vi "Main Tclk.vi"() -> ()   [LabVIEW 2018] (continued)
          tunnel: w2699 -> [w3069 _]
          frame False {
            n3729 = case shown="\"SEM Low Mag Scan\"" w3069 {
              tunnel: w3070 -> [w3073 w3074]
              tunnel: w3071 -> [w3072 w3075]
              frame Default {
                "Detector B" <- w3073
                "Detector A" <- w3072
              }
              frame "SEM Low Mag Scan" {
                "Detector A Low Mag" <- w3075
                "Det A LM" <- w3075
                "Detector B Low Mag" <- w3074
                "Det B LM" <- w3074
              }
            }
          }
          frame True {
            n3730 = shared-variable "My Computer\\Zeiss Library.lvlib\\DetA-scaling"() -> (→"DetA e- Scaling":sgl)  [unwired: 1 in, 1 out]
            n3731 = shared-variable "My Computer\\Zeiss Library.lvlib\\DetB-Scaling"() -> (→"DetB e- Scaling":sgl)  [unwired: 1 in, 1 out]
          }
        }
        n3732 = case shown="False" w2775 {
          tunnel: w2774 -> [w3056 _]
          frame False {
            n3733 = Build Array("Pre image", "Post image") -> (w3058:bool[])
            n3734 = Boolean Array To Number(Boolean array=w3058) -> (number=w3057:u32)
            n3735 = case shown="0, Default" w3057 {
              tunnel: w3056 -> [w3061 w3062 w3063]
              frame 0, Default {
                "FIB Image" <- w3061
              }
              frame 1 {
                "Pre Image" <- w3062
              }
              frame 2 {
                "Post Image" <- w3063
              }
            }
          }
          frame True {
          }
        }
        n3736 = In Range and Coerce(upper limit=w2637, x=w2638, lower limit=sgl 0.0) -> (coerced(x)=w2635:sgl)  [unwired: 1 out]
        n3737 = shared-variable ".\\Zeiss Library.lvlib\\Det"(w2802) -> ()  [unwired: 1 in, 1 out]
        n3738 = Add(x=w2814, y=w2813) -> (x+y=w2812:u16)
        n3739 = Bundle By Name(cluster=w2636, "Focus index stop limit"=w2635) -> (w2634:T36)
        n3740 = Equal To 0?(x=w2812) -> (x = 0?=w2810:bool)
        n3741 = Divide(x=w2715, y=w2711) -> (x/y=w2714:sgl)
        n3742 = Increment(x=w2827) -> (x+1=w2823:sgl)
        n3743 = Divide(x=w2712, y=w2711) -> (x/y=w2713:sgl)
        n3744 = To Double Precision Float(number=w2826) -> (double precision float=w2825:dbl)
        n3745 = Reciprocal(x=w2825) -> (1/x=w2824:dbl)
        n3746 = Multiply(x=w2714, y=w2823) -> (x*y=w2821:sgl)
        n3747 = Multiply(x=w2714, y=w2713) -> (x*y=w2822:sgl)
        n3748 = And(x=w2811, y=w2810) -> (x .and. y?=w2809:bool)
        n3749 = local read "Load recipe"() -> (w2632:bool)
        n3750 = Divide(x=w2822, y=w2623) -> (x/y=w2626:sgl)
        n3751 = Compound Arithmetic op=MULTIPLY(w2629, w2824, w2821, w2713) -> (w2829:dbl)
        "SEM scan time" <- w2829
        n3752 = local read "Detector number"() -> (w2643:i16)
        n3753 = property on="Total pixels recorded" class="Slide (strict)"("Scale.Maximum"=w2626) -> ()  [unwired: 2 in, 2 out]
        n3754 = Quotient & Remainder(x=w2829, y=60.0) -> (x-y*floor(x/y)=w2831:dbl, floor(x/y)=w2832:dbl)
        n3755 = To Variant(anything="FIB Scan Parameters") -> (Variant=w2803:variant)
        n3756 = local read "SEM Status"() -> (w2830:T12)
        n3757 = case shown="Default" w2699 {
          frame "SEM Low Mag Scan" {
          }
          frame Default {
            n3758 = shared-variable ".\\Zeiss Library.lvlib\\Det A Img Tiled"() -> (→"Det A":i16[][])  [unwired: 1 in, 1 out]
            n3759 = shared-variable ".\\Zeiss Library.lvlib\\Det B Img Tiled"() -> (→"Det B":i16[][])  [unwired: 1 in, 1 out]
          }
        }
        n3760 = Bundle By Name(cluster=w2830, "Scan time (s)"=w2831, "Scan time (m)"=w2832, "Detector #"=w2643) -> (w2818:T12)
        n3761 = case shown="False" w2632 {
          tunnel: w2634 -> [_ w2845]
          frame False {
          }
          frame True {
            n3762 = local write "Alert Settings"(w2845) -> ()
          }
        }
        n3763 = shared-variable ".\\Zeiss Library.lvlib\\Realtime Imaging Scan Para"(w2803) -> ()  [unwired: 1 in, 1 out]
        n3764 = To Variant(anything=w2818) -> (Variant=w2817:variant)
        n3765 = case shown="False" w2809 {
          tunnel: w2818 -> [_ w3120]
          tunnel: w2817 -> [_ w3119]
          tunnel: w2807 -> [w3118 _]
          frame False {
            "SEM Status" <- w3118
          }
          frame True {
            n3766 = shared-variable ".\\Zeiss Library.lvlib\\SEMInfo"(w3119) -> ()  [unwired: 2 out]
            n3767 = local write "SEM Status"(w3120) -> ()
          }
        }
        n3768 = local read "Low Mag SEM"() -> (w2670:T30)
        n3769 = local read "SEM Low Mag Scan Parameters"() -> (w2669:T5)
        n3770 = local read "SEM Mid Mag Scan Parameters"() -> (w2668:T5)
        n3771 = Unbundle By Name(w2670) -> ("Low mag scan"=w2753:bool, "Show HM box"=w2773:bool)
        n3772 = property on="Sweep direction" class="Bool (strict)"("Visible"="Sweep enabled") -> ()  [unwired: 2 in, 2 out]
        n3773 = property on="Sweep rate (Hz)" class="DigNum (strict)"("Visible"="Sweep enabled") -> ()  [unwired: 2 in, 2 out]
        n3774 = property on="Level #" class="DigNum (strict)"("Visible"="Sweep enabled") -> ()  [unwired: 2 in, 2 out]
        n3775 = property on="Sweep #" class="DigNum (strict)"("Visible"="Sweep enabled") -> ()  [unwired: 2 in, 2 out]
        n3776 = local read "Milling para"() -> (w2641:T35)
        n3777 = shared-variable ".\\Zeiss Library.lvlib\\FIB PID reset"() -> (w2640:bool)  [unwired: 1 in, 1 out]
        n3778 = local read "Milling para"() -> (w2738:T35)
        n3779 = Unbundle By Name(w2669) -> ("Scan rate (Hz)"=w2671:u32, "X size (um)"=w2675:sgl, "Y size (um)"=w2679:sgl, "Pixel size (nm)"=w2674:sgl)
        n3780 = Unbundle By Name(w2668) -> ("Scan rate (Hz)"=w2741:u32, "X size (um)"=w2709:sgl, "Y size (um)"=w2705:sgl, "Pixel size (nm)"=w2710:sgl)
        n3781 = case shown="False" w2753 {
          tunnel: [T44."Disabled and Grayed Out" ("Disabled") T44."Enabled" ("Disabled")] -> w2772
          tunnel: w2670 -> [w3066 _]
          frame False {
            n3782 = Bundle By Name(cluster=w3066, "Show HM box"=FALSE) -> (w3064:T30)
            n3783 = local write "Low Mag SEM"(w3064) -> ()
          }
          frame True {
          }
        }
        n3784 = property on="Focus (V)" class="DigNum (strict)"("Visible"="Sweep enabled") -> ()  [unwired: 2 in, 2 out]
        n3785 = property on="Angle (V)" class="DigNum (strict)"("Visible"="Sweep enabled") -> ()  [unwired: 2 in, 2 out]
        n3786 = property on="Position (V)" class="DigNum (strict)"("Visible"="Sweep enabled") -> ()  [unwired: 2 in, 2 out]
        n3787 = property on="Imbalance (V)" class="DigNum (strict)"("Visible"="Sweep enabled") -> ()  [unwired: 2 in, 2 out]
        n3788 = Unbundle By Name(w2738) -> ("X offset (um)"=w2780:sgl, "Z offset (um)"=w2781:sgl, "FIB FOV (um)"=w2681:sgl, "Line milling time (s)"=w2794:sgl, "Lines auto pause"=w2770:u16, "FIB PID on"=w2768:bool, "FIB PID measured"=w2718:u8, "FIB PID target"=w2767:sgl, "FIB PID target slope"=w2737:sgl, "FIB PID P"=w2766:sgl, "FIB PID I"=w2765:sgl, "FIB PID D"=w2764:sgl)  [unwired: 1 out]
        "Lines auto pause" <- w2770
        n3789 = Bundle By Name(cluster=w2641, "FIB PID reset"=w2640) -> (w2639:T35)
        n3790 = expression code="x/1000"(w2674) -> (w2678:sgl)
        n3791 = expression code="x/1000"(w2710) -> (w2706:sgl)
        n3792 = expression code="x*4735.8+30400"("Extractor (kV)") -> (w2728:sgl)
        n3793 = expression code="x*4735.8+30420"("Extractor (kV)") -> (w2721:sgl)
        n3794 = To Double Precision Float(number=w2671) -> (double precision float=w2672:dbl)
        n3795 = To Double Precision Float(number=w2741) -> (double precision float=w2740:dbl)
        n3796 = Divide(x=w2675, y=w2678) -> (x/y=w2676:sgl)
        n3797 = Divide(x=w2709, y=w2706) -> (x/y=w2708:sgl)
        n3798 = local write "Milling para"(w2639) -> ()
        n3799 = Reciprocal(x=w2672) -> (1/x=w2673:dbl)
        n3800 = Divide(x=w2679, y=w2678) -> (x/y=w2677:sgl)
        n3801 = Reciprocal(x=w2740) -> (1/x=w2739:dbl)
        n3802 = Divide(x=w2705, y=w2706) -> (x/y=w2707:sgl)
        n3803 = Divide(x=w2780, y=w2681) -> (x/y=w2782:sgl)
        n3804 = Divide(x=w2781, y=w2681) -> (x/y=w2783:sgl)
        n3805 = Compound Arithmetic op=MULTIPLY(w2673, w2676, w2677) -> (→"LM SEM scan time":dbl)
        n3806 = Compound Arithmetic op=MULTIPLY(w2739, w2708, w2707) -> (→"MM SEM scan time":dbl)
        n3807 = Divide(x=w2728, y=w2727) -> (x/y=w2726:sgl)
        n3808 = Divide(x=w2721, y=w2722) -> (x/y=w2723:sgl)
        n3809 = expression code="x*2"(w2782) -> (w2779:sgl)
        n3810 = expression code="x*2"(w2783) -> (w2778:sgl)
        n3811 = Round To Nearest(number=w2726) -> (nearest integer value=w2725:sgl)
        n3812 = Round To Nearest(number=w2723) -> (nearest integer value=w2724:sgl)
        n3813 = shared-variable ".\\Zeiss Library.lvlib\\FIB PID on"(w2768) -> ()  [unwired: 1 in, 1 out]
        n3814 = shared-variable "My Computer\\Zeiss Library.lvlib\\FIB PID measured"(w2718) -> ()  [unwired: 1 in, 1 out]
        n3815 = shared-variable "My Computer\\Zeiss Library.lvlib\\FIB PID target"(w2767) -> ()  [unwired: 1 in, 1 out]
        n3816 = shared-variable "My Computer\\Zeiss Library.lvlib\\FIB PID target slope"(w2737) -> ()  [unwired: 1 in, 1 out]
        n3817 = shared-variable "My Computer\\Zeiss Library.lvlib\\FIB PID-I"(w2765) -> ()  [unwired: 1 in, 1 out]
        n3818 = shared-variable "My Computer\\Zeiss Library.lvlib\\FIB PID-D"(w2764) -> ()  [unwired: 1 in, 1 out]
        n3819 = shared-variable "My Computer\\Zeiss Library.lvlib\\FIB PID-P"(w2766) -> ()  [unwired: 1 in, 1 out]
        n3820 = Multiply(x=w2725, y=w2727) -> (x*y=→"13nA Condenser (V)":sgl)
        n3821 = Multiply(x=w2724, y=w2722) -> (x*y=→"27nA Condenser (V)":sgl)
        n3822 = property on="Show HM box" class="Bool (strict)"("DisabledEnum"=w2772) -> ()  [unwired: 2 in, 2 out]
        n3823 = shared-variable ".\\Zeiss Library.lvlib\\Milling X Offset"(w2779) -> ()  [unwired: 1 in, 1 out]
        n3824 = shared-variable "My Computer\\Zeiss Library.lvlib\\Milling Z Offset"(w2778) -> ()  [unwired: 1 in, 1 out]
        n3825 = shared-variable "My Computer\\Zeiss Library.lvlib\\Line Milling Time (s)"(w2794) -> ()  [unwired: 1 in, 1 out]
        n3826 = shared-variable "My Computer\\Zeiss Library.lvlib\\Milling Lines Auto Pause"(w2770) -> ()  [unwired: 1 in, 1 out]
        n3827 = shared-variable "My Computer\\Zeiss Library.lvlib\\FIB FOV (um)"(w2681) -> ()  [unwired: 1 in, 1 out]
        n3828 = case shown="True" w2773 {
          tunnel: [w3078 w3084] -> w2758
          tunnel: [w3078 w3083] -> w2759
          frame False {
            n3829 = call <vilib>:"Draw Rectangle.vi"("picture"=picture data[5B], "rect"=T47 {"left"=0, "top"=0, "right"=0, "bottom"=0}) -> ("new picture"=w3078:picture)  [unwired: 7 in]
          }
          frame True {
            w3096 = T47 {"left"=0, "top"=0, "right"=0, "bottom"=0} ("rect")
            n3830 = property on="Det A LM" class="IntGraph (strict)"() -> ("Width"=w3110:u32, "Height"=w3114:u32)  [unwired: 2 in, 2 out]
            n3831 = local read "Low Mag SEM"() -> (w3086:T30)
            n3832 = local read "SEM Scan Parameters"() -> (w3111:T26)
            n3833 = property on="Detector A Low Mag" class="IntGraph (strict)"() -> ("Width"=w3090:u32, "Height"=w3089:u32)  [unwired: 2 in, 2 out]
            n3834 = Unbundle By Name(w3086) -> ("Low mag scan FOV (micron)"=w3085:dbl)
            n3835 = Unbundle By Name(w3111) -> ("X center (um)"=w3115:sgl, "Y center (um)"=w3116:sgl, "X size (um)"=w3082:sgl, "Y size (um)"=w3081:sgl)
            n3836 = expression code="x/2"(w3085) -> (w3117:dbl)
            n3837 = Divide(x=w3115, y=w3117) -> (x/y=w3092:dbl)
            n3838 = Divide(x=w3116, y=w3117) -> (x/y=w3088:dbl)
            n3839 = Divide(x=w3082, y=w3117) -> (x/y=w3091:dbl)
            n3840 = Divide(x=w3081, y=w3117) -> (x/y=w3087:dbl)
            n3841 = call "CenterSize to StartEnd or Rect-4C.vi"("Resolution"=w3110, "Size"=w3091, "Center"=w3092) -> ("Rect-4C"=w3113:cluster{"left":i16, "right":i16})  [unwired: 2 in, 2 out]
            n3842 = call "CenterSize to StartEnd or Rect-4C.vi"("Resolution"=w3114, "Size"=w3087, "Center"=w3088) -> ("Rect-4C"=w3112:cluster{"left":i16, "right":i16})  [unwired: 2 in, 2 out]
            n3843 = call "CenterSize to StartEnd or Rect-4C.vi"("Resolution"=w3090, "Size"=w3091, "Center"=w3092) -> ("Rect-4C"=w3097:cluster{"left":i16, "right":i16})  [unwired: 2 in, 2 out]
            n3844 = call "CenterSize to StartEnd or Rect-4C.vi"("Resolution"=w3089, "Size"=w3087, "Center"=w3088) -> ("Rect-4C"=w3098:cluster{"left":i16, "right":i16})  [unwired: 2 in, 2 out]
            n3845 = Unbundle(w3113) -> ("left"=w3107:i16, "right"=w3106:i16)
            n3846 = Unbundle(w3112) -> ("left"=w3105:i16, "right"=w3104:i16)
            n3847 = Unbundle(w3097) -> ("left"=w3099:i16, "right"=w3100:i16)
            n3848 = Unbundle(w3098) -> ("left"=w3101:i16, "right"=w3102:i16)
            n3849 = Bundle By Name(cluster=w3096, "left"=w3107, "right"=w3106, "top"=w3105, "bottom"=w3104) -> (w3103:T47)
            n3850 = Bundle By Name(cluster=w3096, "left"=w3099, "right"=w3100, "top"=w3101, "bottom"=w3102) -> (w3093:T47)
            n3851 = call <vilib>:"Draw Rectangle.vi"("picture"=picture data[5B], "rect"=w3103, "color(black)"=u32 16776960) -> ("new picture"=w3083:picture)  [unwired: 6 in]
            n3852 = call <vilib>:"Draw Rectangle.vi"("picture"=picture data[5B], "rect"=w3093, "color(black)"=u32 16776960) -> ("new picture"=w3084:picture)  [unwired: 6 in]
          }
        }
        n3853 = local read "Focus Index Options"() -> (w2645:T28)
        n3854 = shared-variable ".\\Zeiss Library.lvlib\\Focus Index Array"() -> (w2697:variant)  [unwired: 1 in, 1 out]
        n3855 = shared-variable ".\\Zeiss Library.lvlib\\FIB PID feedback"() -> (→"PID feedback (V)":dbl)  [unwired: 1 in, 1 out]
        n3856 = shared-variable "My Computer\\Zeiss Library.lvlib\\FIB PID feedback mean"() -> (→"PID feedback mean (V)":dbl)  [unwired: 1 in, 1 out]
        n3857 = local read "Alert Settings"() -> (w2736:T36)
        n3858 = shared-variable "My Computer\\Zeiss Library.lvlib\\Focus Index Detector"("FI Detector") -> ()  [unwired: 1 in, 1 out]
        n3859 = Unbundle By Name(w2645) -> ("Show Focus Index"=w2644:bool)
        n3860 = Variant To Data(type="Image Focus Index Array", Variant=w2697) -> (data=w2696:T15, error out=w2692:errorcluster)  [unwired: 1 in]
        n3861 = Unbundle By Name(w2736) -> ("Focus index low limit"=w2735:sgl)
        n3862 = shared-variable ".\\Zeiss Library.lvlib\\Focus Index Array"() -> ()  [unwired: 1 in, 2 out]
        n3863 = call <vilib>:"Clear Errors.vi"("error in (no error)"=w2692) -> ()  [unwired: 5 in, 2 out]
        n3864 = Unbundle By Name(w2692) -> ("status"=w2694:bool)
        n3865 = local read "Focus Index"() -> (w2732:sgl)
        n3866 = Not(x=w2694) -> (.not. x?=w2693:bool)
        n3867 = Compound Arithmetic op=AND(w2644, w2693) -> (w2695:bool)
        n3868 = Greater Or Equal?(x=w2732, y=w2735) -> (x >= y?=w2734:bool)
        n3869 = case shown="True" w2695 {
          tunnel: "FI Detector" -> [_ w3015]
          tunnel: w2696 -> [_ w3014]
          frame False {
            n3870 = call <vilib>:"Draw Rectangle.vi"("picture"=picture data[5B], "rect"=T47 {"left"=0, "top"=0, "right"=0, "bottom"=0}) -> ("new picture"=w3011:picture)  [unwired: 7 in]
            n3871 = property on="Detector A" class="IntGraph (strict)"("PlotImages.Front"=w3011) -> ()  [unwired: 2 in, 2 out]
            n3872 = property on="Detector B" class="IntGraph (strict)"("PlotImages.Front"=w3011) -> ()  [unwired: 2 in, 2 out]
            n3873 = property on="Det A" class="IntGraph (strict)"("PlotImages.Front"=w3011) -> ()  [unwired: 2 in, 2 out]
            n3874 = property on="Det B" class="IntGraph (strict)"("PlotImages.Front"=w3011) -> ()  [unwired: 2 in, 2 out]
          }
          frame True {
            n3875 = stacked-sequence {
              tunnel: w3015 -> [w3035 w3051]
              tunnel: w3014 -> [w3030 _]
              frame #0 {
                n3876 = local read "Focus Index Options"() -> (w3024:T28)
                n3877 = shared-variable ".\\Zeiss Library.lvlib\\Completed tile index"() -> (w3019:u8[])  [unwired: 1 in, 1 out]
                n3878 = local read "Image fit to"() -> (w3016:u8)
                n3879 = shared-variable ".\\Zeiss Library.lvlib\\Y resolution"() -> (w3020:u32)  [unwired: 1 in, 1 out]
                n3880 = shared-variable ".\\Zeiss Library.lvlib\\X resolution"() -> (w3021:u32)  [unwired: 1 in, 1 out]
                n3881 = call <vilib>:"Draw Rectangle.vi"("picture"=picture data[5B], "rect"=T47 {"left"=0, "top"=0, "right"=0, "bottom"=0}) -> ("new picture"=w3028:picture)  [unwired: 7 in]
                n3882 = Unbundle By Name(w3024) -> ("Primary X index"=w3025:u8[][], "Primary Y index"=w3026:u8[][])
                n3883 = case shown="0, Default" w3035 {
                  tunnel: w3030 -> [w3039 w3043]
                  tunnel: [w3038 w3042] -> w3029
                  tunnel: w3028 -> [w3037 w3041]
                  tunnel: [w3036 w3040] -> w3027
                  frame 0, Default {
                    n3884 = Unbundle By Name(w3039) -> ("A Img Focus Index array"=w3038:dbl[][])
                    n3885 = control-ref of="Detector A"() -> (w3036:refnum<vi>)
                    n3886 = property on="Detector B" class="IntGraph (strict)"("PlotImages.Front"=w3037) -> ()  [unwired: 2 in, 2 out]
                  }
                  frame 1 {
                    n3887 = Unbundle By Name(w3043) -> ("B Img Focus Index array"=w3042:dbl[][])
                    n3888 = control-ref of="Detector B"() -> (w3040:refnum<vi>)
                    n3889 = property on="Detector A" class="IntGraph (strict)"("PlotImages.Front"=w3041) -> ()  [unwired: 2 in, 2 out]
                  }
                }
                n3890 = Index Array(array=w3019) -> (element #1=w3018:u8, element #2=w3017:u8)  [unwired: 2 in]
                n3891 = Index Array(array=w3025, index (row)=w3018, index (col)=w3017) -> (element=w3023:u8)
                n3892 = Index Array(array=w3026, index (row)=w3018, index (col)=w3017) -> (element=w3022:u8)
                n3893 = call "Display array on Figure.vi"("Y resolution"=w3020, "X resolution"=w3021, "format string"="%2.3f", "Image fit to"=w3016, "Primary grid @ green"=TRUE, "Input array"=w3029, "Primary Y"=w3022, "Primary X"=w3023, "Image reference"=w3027) -> ()  [unwired: 3 in]
              }
              frame #1 {
                n3894 = local read "SEM Scan Parameters"() -> (w3046:T26)
                n3895 = local read "Focus Index Options"() -> (w3045:T28)
                n3896 = local read "Tiled Image fit to"() -> (w3044:u8)
                n3897 = call <vilib>:"Draw Rectangle.vi"("picture"=picture data[5B], "rect"=T47 {"left"=0, "top"=0, "right"=0, "bottom"=0}) -> ("new picture"=w3048:picture)  [unwired: 7 in]
                n3898 = case shown="0, Default" w3051 {
                  tunnel: w3048 -> [w3053 w3055]
                  tunnel: [w3052 w3054] -> w3047
                  frame 0, Default {
                    n3899 = control-ref of="Det A"() -> (w3052:refnum<vi>)
                    n3900 = property on="Det B" class="IntGraph (strict)"("PlotImages.Front"=w3053) -> ()  [unwired: 2 in, 2 out]
                  }
                  frame 1 {
                    n3901 = control-ref of="Det B"() -> (w3054:refnum<vi>)
                    n3902 = property on="Det A" class="IntGraph (strict)"("PlotImages.Front"=w3055) -> ()  [unwired: 2 in, 2 out]
                  }
                }
                n3903 = call "Display FI locations on tiled image.vi"("Tiled Image fit to"=w3044, "Focus Index Options"=w3045, "SEM Scan Parameters"=w3046, "Image reference"=w3047) -> ()  [unwired: 8 in]
              }
            }
          }
        }
        n3904 = case shown="True" w2734 {
          tunnel: w2732 -> [_ w2958]
          frame False {
          }
          frame True {
            "Last good FI" <- w2958
          }
        }
        n3905 = shared-variable "My Computer\\Zeiss Library.lvlib\\Image Fit to"("Image fit to") -> ()  [unwired: 1 in, 1 out]
        n3906 = case shown="1" "Image fit to" {
          frame 0, Default {
            n3907 = stacked-sequence {
              frame #0 {
                w2896 = u8 0 ("Y Scale.Scale Fit")
                w2897 = u8 1 ("X Scale.Scale Fit")
                n3908 = property on="Detector A" class="IntGraph (strict)"("XScale.ScaleFit"=w2897) -> ()  [unwired: 2 in, 2 out]
                n3909 = property on="Detector A" class="IntGraph (strict)"("YScale.ScaleFit"=w2896) -> ()  [unwired: 2 in, 2 out]
                n3910 = property on="Detector B" class="IntGraph (strict)"("XScale.ScaleFit"=w2897) -> ()  [unwired: 2 in, 2 out]
                n3911 = property on="Detector B" class="IntGraph (strict)"("YScale.ScaleFit"=w2896) -> ()  [unwired: 2 in, 2 out]
              }
              frame #1 {
                n3912 = property on="Detector A" class="IntGraph (strict)"() -> ("XScale.Maximum"=w2899:dbl)  [unwired: 2 in, 2 out]
                n3913 = property on="Detector B" class="IntGraph (strict)"() -> ("XScale.Maximum"=w2898:dbl)  [unwired: 2 in, 2 out]
                n3914 = property on="Detector A" class="IntGraph (strict)"("YScale.Maximum"=w2899) -> ()  [unwired: 2 in, 2 out]
                n3915 = property on="Detector B" class="IntGraph (strict)"("YScale.Maximum"=w2898) -> ()  [unwired: 2 in, 2 out]
              }
            }
          }
          frame 1 {
            n3916 = stacked-sequence {
              frame #0 {
                w2900 = u8 1 ("Y Scale.Scale Fit")
                w2901 = u8 0 ("X Scale.Scale Fit")
                n3917 = property on="Detector A" class="IntGraph (strict)"("XScale.ScaleFit"=w2901) -> ()  [unwired: 2 in, 2 out]
                n3918 = property on="Detector A" class="IntGraph (strict)"("YScale.ScaleFit"=w2900) -> ()  [unwired: 2 in, 2 out]
                n3919 = property on="Detector B" class="IntGraph (strict)"("XScale.ScaleFit"=w2901) -> ()  [unwired: 2 in, 2 out]
                n3920 = property on="Detector B" class="IntGraph (strict)"("YScale.ScaleFit"=w2900) -> ()  [unwired: 2 in, 2 out]
              }
              frame #1 {
                n3921 = property on="Detector A" class="IntGraph (strict)"() -> ("YScale.Maximum"=w2903:dbl)  [unwired: 2 in, 2 out]
                n3922 = property on="Detector B" class="IntGraph (strict)"() -> ("YScale.Maximum"=w2902:dbl)  [unwired: 2 in, 2 out]
                n3923 = property on="Detector A" class="IntGraph (strict)"("XScale.Maximum"=w2903) -> ()  [unwired: 2 in, 2 out]
                n3924 = property on="Detector B" class="IntGraph (strict)"("XScale.Maximum"=w2902) -> ()  [unwired: 2 in, 2 out]
              }
            }
          }
        }
        n3925 = local read "Mid Mag SEM"() -> (w2680:T29)
        n3926 = Unbundle By Name(w2680) -> ("Mid mag scan"=w2755:bool, "Show MM box"=w2756:bool)
        n3927 = local read "Image Tabs"() -> (w2730:T37)
        n3928 = And(x=w2753, y=w2755) -> (x .and. y?=w2754:bool)
        n3929 = case shown="\"All\"" w2730 {
          frame "All" {
            w2937 = FALSE ("Visible")
            n3930 = property on="Image fit to" class="Ring (strict)"("Visible"=w2937) -> ()  [unwired: 2 in, 2 out]
            n3931 = property on="Milling Z realtime (V)" class="DigNum (strict)"("Visible"=w2937) -> ()  [unwired: 2 in, 2 out]
          }
          frame "Detector A", Default {
            n3932 = property on="Image fit to" class="Ring (strict)"("Visible"=TRUE) -> ()  [unwired: 2 in, 2 out]
            n3933 = property on="Milling Z realtime (V)" class="DigNum (strict)"("Visible"=FALSE) -> ()  [unwired: 2 in, 2 out]
          }
          frame "Detector B" {
            n3934 = property on="Image fit to" class="Ring (strict)"("Visible"=TRUE) -> ()  [unwired: 2 in, 2 out]
            n3935 = property on="Milling Z realtime (V)" class="DigNum (strict)"("Visible"=FALSE) -> ()  [unwired: 2 in, 2 out]
          }
          frame "Detector A Low Mag" {
            w2942 = FALSE ("Visible")
            n3936 = property on="Image fit to" class="Ring (strict)"("Visible"=w2942) -> ()  [unwired: 2 in, 2 out]
            n3937 = property on="Milling Z realtime (V)" class="DigNum (strict)"("Visible"=w2942) -> ()  [unwired: 2 in, 2 out]
          }
          frame "Detector B Low Mag" {
            w2943 = FALSE ("Visible")
            n3938 = property on="Image fit to" class="Ring (strict)"("Visible"=w2943) -> ()  [unwired: 2 in, 2 out]
            n3939 = property on="Milling Z realtime (V)" class="DigNum (strict)"("Visible"=w2943) -> ()  [unwired: 2 in, 2 out]
          }
          frame "FIB" {
            n3940 = property on="Image fit to" class="Ring (strict)"("Visible"=FALSE) -> ()  [unwired: 2 in, 2 out]
            n3941 = property on="Milling Z realtime (V)" class="DigNum (strict)"("Visible"=TRUE) -> ()  [unwired: 2 in, 2 out]
          }
          frame "FIB Milling Offset after Pause" {
            w2946 = FALSE ("Visible")
            n3942 = property on="Image fit to" class="Ring (strict)"("Visible"=w2946) -> ()  [unwired: 2 in, 2 out]
            n3943 = property on="Milling Z realtime (V)" class="DigNum (strict)"("Visible"=w2946) -> ()  [unwired: 2 in, 2 out]
          }
          frame "Auto Focus / Stig / Align" {
            w2947 = FALSE ("Visible")
            n3944 = property on="Image fit to" class="Ring (strict)"("Visible"=w2947) -> ()  [unwired: 2 in, 2 out]
            n3945 = property on="Milling Z realtime (V)" class="DigNum (strict)"("Visible"=w2947) -> ()  [unwired: 2 in, 2 out]
          }
          frame "Imaging Quality" {
            w2948 = FALSE ("Visible")
            n3946 = property on="Image fit to" class="Ring (strict)"("Visible"=w2948) -> ()  [unwired: 2 in, 2 out]
            n3947 = property on="Milling Z realtime (V)" class="DigNum (strict)"("Visible"=w2948) -> ()  [unwired: 2 in, 2 out]
          }
          frame "Temp. and Currents" {
            w2949 = FALSE ("Visible")
            n3948 = property on="Image fit to" class="Ring (strict)"("Visible"=w2949) -> ()  [unwired: 2 in, 2 out]
            n3949 = property on="Milling Z realtime (V)" class="DigNum (strict)"("Visible"=w2949) -> ()  [unwired: 2 in, 2 out]
          }
          frame "FIB HV Data" {
            w2950 = FALSE ("Visible")
            n3950 = property on="Image fit to" class="Ring (strict)"("Visible"=w2950) -> ()  [unwired: 2 in, 2 out]
            n3951 = property on="Milling Z realtime (V)" class="DigNum (strict)"("Visible"=w2950) -> ()  [unwired: 2 in, 2 out]
          }
          frame "Logging: Realtime Graphs" {
            n3952 = property on="Image fit to" class="Ring (strict)"("Visible"=FALSE) -> ()  [unwired: 2 in, 2 out]
            n3953 = property on="Milling Z realtime (V)" class="DigNum (strict)"("Visible"=TRUE) -> ()  [unwired: 2 in, 2 out]
          }
        }
        n3954 = case shown="False" w2754 {
          tunnel: [T44."Disabled and Grayed Out" ("Disabled") T44."Enabled" ("Disabled")] -> w2757
          tunnel: w2680 -> [w2969 _]
          frame False {
            n3955 = Bundle By Name(cluster=w2969, "Show MM box"=FALSE ("Show HM box")) -> (w2968:T29)
            n3956 = local write "Mid Mag SEM"(w2968) -> ()
          }
          frame True {
          }
        }
        n3957 = local read "Load recipe"() -> (w2700:bool)
        n3958 = property on="Show MM box" class="Bool (strict)"("DisabledEnum"=w2757) -> ()  [unwired: 2 in, 2 out]
        n3959 = case shown="False" w2700 {
          frame False {
            n3960 = local read "X shift (nm/image)"() -> (w2934:sgl)
            n3961 = local read "Y shift (nm/image)"() -> (w2935:sgl)
            n3962 = local read "SEM Scan Parameters"() -> (w2926:T26)
            n3963 = local read "Detector Information"() -> (w2907:T8)
            n3964 = local read "SEM Options"() -> (w2925:T27)
            n3965 = local read "Focus Index Options"() -> (w2906:T28)
            n3966 = local read "Image fit to"() -> (w2911:u8)
            n3967 = local read "File Information"() -> (w2924:T31)
            n3968 = local read "Low Mag SEM"() -> (w2923:T30)
            n3969 = local read "Mid Mag SEM"() -> (w2917:T29)
            n3970 = local read "FIB-SEM Angle"() -> (w2922:dbl)
            n3971 = local read "Milling para"() -> (w2921:T35)
            n3972 = local read "FI Detector"() -> (w2927:u16)
            n3973 = local read "Auto Optimzation"() -> (w2928:bool)
            n3974 = local read "Images per Auto Optimization"() -> (w2929:u16)
            n3975 = local read "AF Range (nm)"() -> (w2930:sgl)
            n3976 = local read "AF Steps"() -> (w2931:u8)
            n3977 = local read "AS Range (%)"() -> (w2932:sgl)
            n3978 = local read "AS Steps"() -> (w2933:u8)
            n3979 = local read "AA Range (%)"() -> (w2913:sgl)
            n3980 = local read "AA Steps"() -> (w2912:u8)
            n3981 = local read "FIB Y zoom pixel (nm)"() -> (w2920:dbl)
            n3982 = local read "Mail server"() -> (w2919:string)
            n3983 = local read "Email Alert Recipients"() -> (w2918:string[])
            n3984 = local read "Alert Settings"() -> (w2916:T36)
            n3985 = local read "Reheat Parameters"() -> (w2910:T1)
            n3986 = local read "Start FIB HV DataLog"() -> (w2909:bool)
            n3987 = local read "Interval (s)"() -> (w2908:u16)
            n3988 = Bundle By Name(cluster="Recipe input", "SEM Scan Parameters"=w2926, "Detector Information"=w2907, "SEM Options"=w2925, "Focus Index Options"=w2906, "Image fit to"=w2911, "File Information"=w2924, "Low mag SEM"=w2923, "Mid Mag SEM"=w2917, "FIB-SEM Angle"=w2922, "Milling para"=w2921, "FI Detector"=w2927, "Auto Optimzation"=w2928, "Images per Auto Optimization"=w2929, "AF Range (nm)"=w2930, "AF Steps"=w2931, "AS Range (%)"=w2932, "AS Steps"=w2933, "AA Range (%)"=w2913, "AA Steps"=w2912, "X shift (nm/frame)"=w2934, "Y shift (nm/frame)"=w2935, "FIB Y zoom pixel (nm)"=w2920, "Mail server"=w2919, "Email Alert Recipents"=w2918, "Alert Settings"=w2916, "Reheat Parameters"=w2910, "Start FIB HV DataLog"=w2909, "Interval (s)"=w2908) -> (w2915:T7)
            n3989 = To Variant(anything=w2915) -> (Variant=w2914:variant)
            n3990 = shared-variable ".\\Zeiss Library.lvlib\\Recipe input"(w2914) -> ()  [unwired: 1 in, 1 out]
            n3991 = local write "Recipe input"(w2915) -> ()
          }
          frame True {
          }
        }
        n3992 = case shown="True" w2756 {
          tunnel: w2759 -> [w2973 w2979]
          tunnel: w2758 -> [w2972 w2977]
          tunnel: [w2973 w2978] -> w2747
          tunnel: [w2972 w2976] -> w2746
          frame False {
          }
          frame True {
            w2990 = T47 {"left"=0, "top"=0, "right"=0, "bottom"=0} ("rect")
            n3993 = property on="Det A LM" class="IntGraph (strict)"() -> ("Width"=w3003:u32, "Height"=w3007:u32)  [unwired: 2 in, 2 out]
            n3994 = local read "Low Mag SEM"() -> (w2981:T30)
            n3995 = local read "Mid Mag SEM"() -> (w3004:T29)
            n3996 = property on="Detector A Low Mag" class="IntGraph (strict)"() -> ("Width"=w2985:u32, "Height"=w2984:u32)  [unwired: 2 in, 2 out]
            n3997 = Unbundle By Name(w2981) -> ("Low mag scan FOV (micron)"=w2980:dbl)
            n3998 = Unbundle By Name(w3004) -> ("X center (um)"=w3008:dbl, "Y center (um)"=w3009:dbl, "X size (um)"=w2975:sgl, "Y size (um)"=w2974:sgl)
            n3999 = expression code="x/2"(w2980) -> (w3010:dbl)
            n4000 = Divide(x=w3008, y=w3010) -> (x/y=w2987:dbl)
            n4001 = Divide(x=w3009, y=w3010) -> (x/y=w2983:dbl)
            n4002 = Divide(x=w2975, y=w3010) -> (x/y=w2986:dbl)
            n4003 = Divide(x=w2974, y=w3010) -> (x/y=w2982:dbl)
            n4004 = call "CenterSize to StartEnd or Rect-4C.vi"("Resolution"=w3003, "Size"=w2986, "Center"=w2987) -> ("Rect-4C"=w3006:cluster{"left":i16, "right":i16})  [unwired: 2 in, 2 out]
            n4005 = call "CenterSize to StartEnd or Rect-4C.vi"("Resolution"=w3007, "Size"=w2982, "Center"=w2983) -> ("Rect-4C"=w3005:cluster{"left":i16, "right":i16})  [unwired: 2 in, 2 out]
            n4006 = call "CenterSize to StartEnd or Rect-4C.vi"("Resolution"=w2985, "Size"=w2986, "Center"=w2987) -> ("Rect-4C"=w2991:cluster{"left":i16, "right":i16})  [unwired: 2 in, 2 out]
            n4007 = call "CenterSize to StartEnd or Rect-4C.vi"("Resolution"=w2984, "Size"=w2982, "Center"=w2983) -> ("Rect-4C"=w2992:cluster{"left":i16, "right":i16})  [unwired: 2 in, 2 out]
            n4008 = Unbundle(w3006) -> ("left"=w3001:i16, "right"=w3000:i16)
            n4009 = Unbundle(w3005) -> ("left"=w2999:i16, "right"=w2998:i16)
            n4010 = Unbundle(w2991) -> ("left"=w2993:i16, "right"=w2994:i16)
            n4011 = Unbundle(w2992) -> ("left"=w2995:i16, "right"=w2996:i16)
            n4012 = Bundle By Name(cluster=w2990, "left"=w3001, "right"=w3000, "top"=w2999, "bottom"=w2998) -> (w2997:T47)
            n4013 = Bundle By Name(cluster=w2990, "left"=w2993, "right"=w2994, "top"=w2995, "bottom"=w2996) -> (w2988:T47)
            n4014 = call <vilib>:"Draw Rectangle.vi"("picture"=w2979, "rect"=w2997, "color(black)"=u32 3381759) -> ("new picture"=w2978:picture)  [unwired: 6 in]
            n4015 = call <vilib>:"Draw Rectangle.vi"("picture"=w2977, "rect"=w2988, "color(black)"=u32 3381759) -> ("new picture"=w2976:picture)  [unwired: 6 in]
          }
        }
        n4016 = call <vilib>:"Draw Rectangle.vi"("picture"=picture data[5B], "rect"=T47 {"left"=0, "top"=0, "right"=0, "bottom"=0}) -> ("new picture"=w2743:picture)  [unwired: 7 in]
        n4017 = local read "SEM Options"() -> (w2760:T27)
        n4018 = local read "Hardware Configuration"() -> (w2689:T25)
        n4019 = Unbundle By Name(w2689) -> ("Brightness A"=w2688:dbl, "Contrast A"=w2687:dbl, "Detector B name"=w2686:string, "Brightness B"=w2685:dbl, "Contrast B"=w2684:dbl)
        n4020 = local read "Machine Type"() -> (w2657:u8)
        n4021 = local read "SEM Scan Parameters"() -> (w2665:T26)
        n4022 = local read "SEM scan time"() -> (w2628:dbl)
        n4023 = local read "Milling time (s)"() -> (w2661:sgl)
        n4024 = local read "SEM-FIB Delay (s)"() -> (w2622:u32)
        n4025 = local read "Focus Index Options"() -> (w2646:T28)
        n4026 = Unbundle By Name(w2760) -> ("Detector A"=w2762:bool, "Detector B"=w2763:bool)
        n4027 = Bundle By Name(cluster="Detector Information", "Brightness A"=w2688, "Contrast A"=w2687, "Detector B name"=w2686, "Brightness B"=w2685, "Contrast B"=w2684) -> (w2682:T8)
        n4028 = case shown="2" w2657 {
          tunnel: [u8 3 ("x*y") u8 3 ("x*y") u8 2 ("x*y")] -> w2656
          frame 0, Default {
          }
          frame 1 {
          }
          frame 2 {
          }
        }
        n4029 = Unbundle By Name(w2665) -> ("X tiles"=w2663:u8, "Y tiles"=w2666:u8)
        n4030 = Build Array(w2762, w2763) -> (w2761:bool[])
        n4031 = Unbundle By Name(w2646) -> ("Focus Index primary grid center"=w2651:bool, "X Grids"=w2650:u8[][], "Primary X index"=w2649:u8[][], "Y Grids"=w2648:u8[][], "Primary Y index"=w2647:u8[][])
        n4032 = Boolean Array To Number(Boolean array=w2761) -> (number=w2745:u32)
        n4033 = Multiply(x=w2663, y=w2666) -> (x*y=w2660:u8)
        n4034 = Decrement(x=w2660) -> (x-1=w2659:u8)
        n4035 = local write "Detector Information"(w2682) -> ()
        n4036 = Multiply(x=w2656, y=w2659) -> (x*y=w2658:u8)
        n4037 = case shown="1, Default" w2745 {
          tunnel: w2747 -> [w2961 w2964 w2966]
          tunnel: w2746 -> [w2960 w2963 w2965]
          tunnel: [w2959 w2964 w2966] -> w2748
          tunnel: [w2961 w2962 w2966] -> w2749
          tunnel: [w2960 w2962 w2965] -> w2750
          tunnel: [w2959 w2963 w2965] -> w2751
          tunnel: w2743 -> [w2959 w2962 _]
          frame 1, Default {
          }
          frame 2 {
          }
          frame 3 {
          }
        }
        n4038 = local read "Overhead (s)"() -> (w2662:sgl)
        n4039 = property on="Det A LM" class="IntGraph (strict)"("PlotImages.Front"=w2749) -> ()  [unwired: 2 in, 2 out]
        n4040 = property on="Det B LM" class="IntGraph (strict)"("PlotImages.Front"=w2748) -> ()  [unwired: 2 in, 2 out]
        n4041 = property on="Detector A Low Mag" class="IntGraph (strict)"("PlotImages.Front"=w2750) -> ()  [unwired: 2 in, 2 out]
        n4042 = property on="Detector B Low Mag" class="IntGraph (strict)"("PlotImages.Front"=w2751) -> ()  [unwired: 2 in, 2 out]
        n4043 = case shown="False" w2651 {
          tunnel: w2650 -> [w2850 w2871]
          tunnel: w2649 -> [w2849 _]
          tunnel: w2648 -> [w2848 w2870]
          tunnel: w2647 -> [w2847 _]
          tunnel: w2646 -> [w2846 w2869]
          frame False {
            n4044 = for {
              tunnel: w2850 -> [w2861] mode=indexing
              tunnel: w2849 -> [w2860] mode=indexing
              tunnel: [w2859] -> w2854 mode=indexing
              tunnel: w2848 -> [w2858] mode=indexing
              tunnel: w2847 -> [w2857] mode=indexing
              tunnel: [w2856] -> w2853 mode=indexing
              tunnel: u8 1 ("x") -> [w2855]
              n4045 = for {
                tunnel: w2861 -> [w2868] mode=indexing
                tunnel: w2860 -> [w2867] mode=indexing
                tunnel: [w2866] -> w2859 mode=indexing
                tunnel: w2858 -> [w2865] mode=indexing
                tunnel: w2857 -> [w2864] mode=indexing
                tunnel: [w2863] -> w2856 mode=indexing
                tunnel: w2855 -> [w2862]
                n4046 = In Range and Coerce(upper limit=w2868, x=w2867, lower limit=w2862) -> (coerced(x)=w2866:u8)  [unwired: 1 out]
                n4047 = In Range and Coerce(upper limit=w2865, x=w2864, lower limit=w2862) -> (coerced(x)=w2863:u8)  [unwired: 1 out]
              }
            }
            n4048 = Bundle By Name(cluster=w2846, "Primary X index"=w2854, "Primary Y index"=w2853) -> (w2852:T28)
            n4049 = local write "Focus Index Options"(w2852) -> ()
          }
          frame True {
            n4050 = for {
              tunnel: w2871 -> [w2882] mode=indexing
              tunnel: w2870 -> [w2881] mode=indexing
              tunnel: [w2880] -> w2875 mode=indexing
              tunnel: [w2879] -> w2874 mode=indexing
              tunnel: [w2878] -> w2873 mode=indexing
              tunnel: [w2877] -> w2872 mode=indexing
              n4051 = for {
                tunnel: w2882 -> [w2888] mode=indexing
                tunnel: w2881 -> [w2887] mode=indexing
                tunnel: [w2886] -> w2880 mode=indexing
                tunnel: [w2885] -> w2879 mode=indexing
                tunnel: [w2884] -> w2878 mode=indexing
                tunnel: [w2883] -> w2877 mode=indexing
                n4052 = To Single Precision Float(number=w2888) -> (single precision float=w2891:sgl)
                n4053 = To Single Precision Float(number=w2887) -> (single precision float=w2890:sgl)
                n4054 = expression code="x/2"(w2891) -> (w2892:sgl)
                n4055 = expression code="x/2"(w2890) -> (w2889:sgl)
                n4056 = Round Toward +Infinity(x=w2892) -> (ceil(x): smallest int >= x=w2885:sgl)
                n4057 = Round Toward +Infinity(x=w2889) -> (ceil(x): smallest int >= x=w2883:sgl)
                n4058 = expression code="x*2-1"(w2885) -> (w2886:sgl)
                n4059 = expression code="x*2-1"(w2883) -> (w2884:sgl)
              }
            }
            n4060 = Bundle By Name(cluster=w2869, "X Grids"=w2875, "Primary X index"=w2874, "Y Grids"=w2873, "Primary Y index"=w2872) -> (w2876:T28)
            n4061 = local write "Focus Index Options"(w2876) -> ()
          }
        }
        n4062 = local read "SEM Options"() -> (w2731:T27)
        n4063 = local read "SEM Parameters"() -> (w2834:T13)
        n4064 = local read "Detector Information"() -> (w2833:T8)
        n4065 = Compound Arithmetic op=ADD(w2662, w2658, w2628, w2661, w2622) -> (→"Est. cycle time (s)":dbl)
        n4066 = shared-variable "My Computer\\Zeiss Library.lvlib\\Milling Post-pause Lines"() -> (→"Rect Milling Post-pause Lines":u16)  [unwired: 1 in, 1 out]
        n4067 = shared-variable ".\\Zeiss Library.lvlib\\Realtime Imaging Info"() -> (w2801:variant)  [unwired: 1 in, 1 out]
        n4068 = shared-variable ".\\Zeiss Library.lvlib\\Milling Progress"() -> (w2800:u8[])  [unwired: 1 in, 1 out]
        n4069 = local read "SEM Status"() -> (w2704:T12)
        n4070 = Unbundle By Name(w2731) -> ("8-bit"=w2652:bool, "Inverse A"=w2820:bool, "Inverse B"=w2804:bool)
        n4071 = Unbundle By Name(w2834) -> ("Detector A"=w2839:string)
        n4072 = Unbundle By Name(w2833) -> ("Detector B name"=w2840:string)
        n4073 = Unbundle By Name(w2704) -> ("Y tile"=w2703:u8, "X tile"=w2702:u8)
        n4074 = property on="DetA e- Scaling" class="DigNum (strict)"("Visible"=w2652) -> ()  [unwired: 2 in, 2 out]
        n4075 = Select(t=u32[] [16448250, 16711422, 16645629, 16579836, 16514043, 16448250, 16382457, 16316664, 16250871, 16185078, 16119285, 16053492, 15987699, 15921906, 15856113, 15790320, 15724527, 15658734, 15592941, 15527148, 15461355, 15395562, 15329769, 15263976, 15198183, 15132390, 15066597, 15000804, 14935011, 14869218, 14803425, 14737632, 14671839, 14606046, 14540253, 14474460, 14408667, 14342874, 14277081, 14211288, 14145495, 14079702, 14013909, 13948116, 13882323, 13816530, 13750737, 13684944, 13619151, 13553358, 13487565, 13421772, 13355979, 13290186, 13224393, 13158600, 13092807, 13027014, 12961221, 12895428, 12829635, 12763842, 12698049, 12632256, 12566463, 12500670, 12434877, 12369084, 12303291, 12237498, 12171705, 12105912, 12040119, 11974326, 11908533, 11842740, 11776947, 11711154, 11645361, 11579568, 11513775, 11447982, 11382189, 11316396, 11250603, 11184810, 11119017, 11053224, 10987431, 10921638, 10855845, 10790052, 10724259, 10658466, 10592673, 10526880, 10461087, 10395294, 10329501, 10263708, 10197915, 10132122, 10066329, 10000536, 9934743, 9868950, 9803157, 9737364, 9671571, 9605778, 9539985, 9474192, 9408399, 9342606, 9276813, 9211020, 9145227, 9079434, 9013641, 8947848, 8882055, 8816262, 8750469, 8684676, 8618883, 8553090, 8487297, 8421504, 8355711, 8289918, 8224125, 8158332, 8092539, 8026746, 7960953, 7895160, 7829367, 7763574, 7697781, 7631988, 7566195, 7500402, 7434609, 7368816, 7303023, 7237230, 7171437, 7105644, 7039851, 6974058, 6908265, 6842472, 6776679, 6710886, 6645093, 6579300, 6513507, 6447714, 6381921, 6316128, 6250335, 6184542, 6118749, 6052956, 5987163, 5921370, 5855577, 5789784, 5723991, 5658198, 5592405, 5526612, 5460819, 5395026, 5329233, 5263440, 5197647, 5131854, 5066061, 5000268, 4934475, 4868682, 4802889, 4737096, 4671303, 4605510, 4539717, 4473924, 4408131, 4342338, 4276545, 4210752, 4144959, 4079166, 4013373, 3947580, 3881787, 3815994, 3750201, 3684408, 3618615, 3552822, 3487029, 3421236, 3355443, 3289650, 3223857, 3158064, 3092271, 3026478, 2960685, 2894892, 2829099, 2763306, 2697513, 2631720, 2565927, 2500134, 2434341, 2368548, 2302755, 2236962, 2171169, 2105376, 2039583, 1973790, 1907997, 1842204, 1776411, 1710618, 1644825, 1579032, 1513239, 1447446, 1381653, 1315860, 1250067, 1184274, 1118481, 1052688, 986895, 921102, 855309, 789516, 723723, 657930, 592137, 526344, 460551, 394758, 328965, 263172, 197379, 131586, 65793, 16777222] ("256 gray scale inverse"), s=w2820, f=u32[] [16777222, 65793, 131586, 197379, 263172, 328965, 394758, 460551, 526344, 592137, 657930, 723723, 789516, 855309, 921102, 986895, 1052688, 1118481, 1184274, 1250067, 1315860, 1381653, 1447446, 1513239, 1579032, 1644825, 1710618, 1776411, 1842204, 1907997, 1973790, 2039583, 2105376, 2171169, 2236962, 2302755, 2368548, 2434341, 2500134, 2565927, 2631720, 2697513, 2763306, 2829099, 2894892, 2960685, 3026478, 3092271, 3158064, 3223857, 3289650, 3355443, 3421236, 3487029, 3552822, 3618615, 3684408, 3750201, 3815994, 3881787, 3947580, 4013373, 4079166, 4144959, 4210752, 4276545, 4342338, 4408131, 4473924, 4539717, 4605510, 4671303, 4737096, 4802889, 4868682, 4934475, 5000268, 5066061, 5131854, 5197647, 5263440, 5329233, 5395026, 5460819, 5526612, 5592405, 5658198, 5723991, 5789784, 5855577, 5921370, 5987163, 6052956, 6118749, 6184542, 6250335, 6316128, 6381921, 6447714, 6513507, 6579300, 6645093, 6710886, 6776679, 6842472, 6908265, 6974058, 7039851, 7105644, 7171437, 7237230, 7303023, 7368816, 7434609, 7500402, 7566195, 7631988, 7697781, 7763574, 7829367, 7895160, 7960953, 8026746, 8092539, 8158332, 8224125, 8289918, 8355711, 8421504, 8487297, 8553090, 8618883, 8684676, 8750469, 8816262, 8882055, 8947848, 9013641, 9079434, 9145227, 9211020, 9276813, 9342606, 9408399, 9474192, 9539985, 9605778, 9671571, 9737364, 9803157, 9868950, 9934743, 10000536, 10066329, 10132122, 10197915, 10263708, 10329501, 10395294, 10461087, 10526880, 10592673, 10658466, 10724259, 10790052, 10855845, 10921638, 10987431, 11053224, 11119017, 11184810, 11250603, 11316396, 11382189, 11447982, 11513775, 11579568, 11645361, 11711154, 11776947, 11842740, 11908533, 11974326, 12040119, 12105912, 12171705, 12237498, 12303291, 12369084, 12434877, 12500670, 12566463, 12632256, 12698049, 12763842, 12829635, 12895428, 12961221, 13027014, 13092807, 13158600, 13224393, 13290186, 13355979, 13421772, 13487565, 13553358, 13619151, 13684944, 13750737, 13816530, 13882323, 13948116, 14013909, 14079702, 14145495, 14211288, 14277081, 14342874, 14408667, 14474460, 14540253, 14606046, 14671839, 14737632, 14803425, 14869218, 14935011, 15000804, 15066597, 15132390, 15198183, 15263976, 15329769, 15395562, 15461355, 15527148, 15592941, 15658734, 15724527, 15790320, 15856113, 15921906, 15987699, 16053492, 16119285, 16185078, 16250871, 16316664, 16382457, 16448250, 16514043, 16579836, 16645629, 16711422, 16448250] ("256 gray scale")) -> (s? t:f=w2806:u32[])
        n4076 = Variant To Data(Variant=w2801) -> (data=→"FIB Status":T20)  [unwired: 2 in, 1 out]
        n4077 = Index Array(array=w2800) -> (element #1=→"Line progress":u8, element #2=→"Total\nprogress":u8)  [unwired: 2 in]
        n4078 = Build Array(w2703, w2702) -> (w2701:u8[])
        n4079 = property on="Detector A" class="IntGraph (strict)"("Color Table"=w2806, "Caption.Text"=w2839) -> ()  [unwired: 2 in, 2 out]
